vi "WASH log error file.vi"(5 "Time Stamp":timestamp, 7 "error levels":T1, 8 "error in (no error)":errorcluster, 9 "step name":string, 10 "station name":string, 11 "refnum out":refnum<file>) -> (0 "error out":errorcluster)   [LabVIEW 2012]
doc: "Saves data to the error log file.\n\n[Covers: EH2]\n[Covers: EH2A]\n[Covers: EH2B]\n[Covers: EH2C]\n[Covers: EH2D]"
uses:
  type defs/WASH error levels.ctl
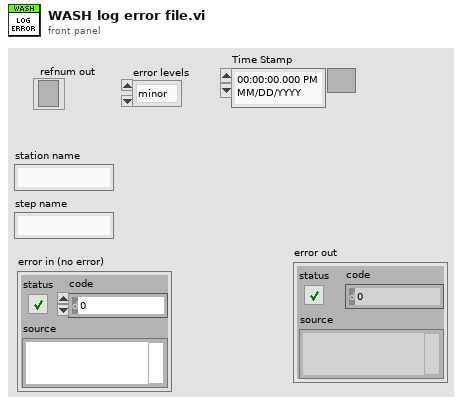
[diagram p1: front panel]
types:
  T1 = typedef "WASH error levels.ctl" = enum16{"minor", "wash cycle", "system"}
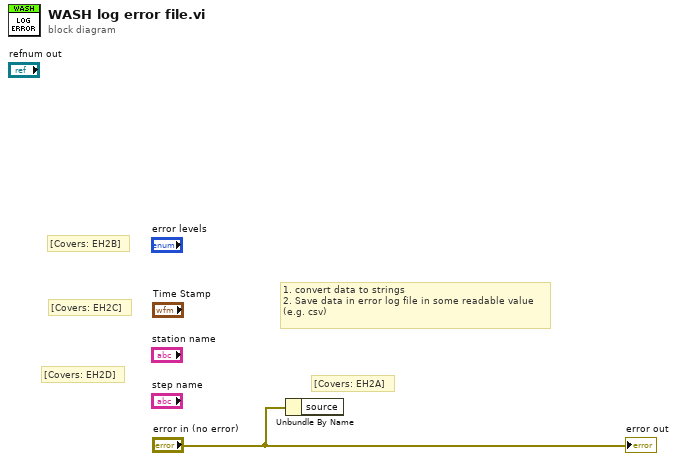
[diagram p0: block diagram]
diagram:
  # "[Covers: EH2D]"
  # "[Covers: EH2C]"
  # "[Covers: EH2B]"
  # "[Covers: EH2A]"
  # "1. convert data to strings\n2. Save data in error log file in some readable value\n(e.g. csv)"
  n1 = Unbundle By Name("error in (no error)") -> ()  [unwired: 1 out]
  "error out" <- "error in (no error)"
